vi "getnumber.vi"(3 "High Limit":dbl=5.0 format="%.2f", 5 "Low Limit":dbl=3.0 format="%.2f") -> (1 "Random Number within Limits":dbl format="%.2f")   [LabVIEW 2011]
doc: "Returns a random number within the specified limits"
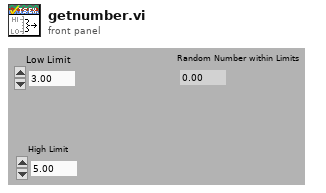
[diagram p1: front panel]
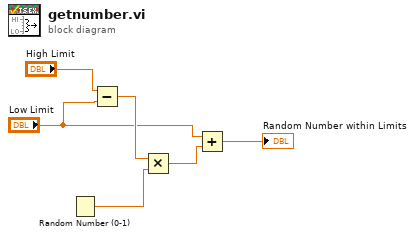
[diagram p0: block diagram]
diagram:
  n1 = Random Number (0-1)() -> (number: 0 to 1=w4:dbl)
  n2 = Subtract(x="High Limit", y="Low Limit") -> (x-y=w2:dbl)
  n3 = Multiply(x=w2, y=w4) -> (x*y=w5:dbl)
  n4 = Add(x="Low Limit", y=w5) -> (x+y=→"Random Number within Limits":dbl)
